vi "PositionCtrl_TurnToAngle_Example.vi"() -> ()   [LabVIEW 2019]
uses:
  <vilib>/Rock Robotics/WPI/ThirdParty/JAS_Junk/TrajLib/SlewRateLimiter_New.vi
  <vilib>/Rock Robotics/WPI/ThirdParty/JAS_Junk/TrajLib/SlewRateLimiter_Reset.vi
  <vilib>/Rock Robotics/WPI/ThirdParty/JAS_Junk/TrajLib/SlewRateLimiter_Calculate.vi
  <vilib>/Rock Robotics/WPI/ThirdParty/JAS_Junk/TrajLib/SlewRateLimiter_SetRate.vi
  <vilib>/Rock Robotics/WPI/ThirdParty/JAS_Junk/TrajLib/Util_GetTime.vi
  <vilib>/Rock Robotics/WPI/ThirdParty/JAS_Junk/TrajLib/VI/Util_GetTime_U32.vi
  <vilib>/Rock Robotics/WPI/ThirdParty/JAS_Junk/TrajLib/VI/Util_GetTime_U64.vi
  <vilib>/Rock Robotics/WPI/ThirdParty/JAS_Junk/TrajLib/Trajectory_Library.lvlib
panel:
  in  "Tab Control":enum32{"Operation", "Tuning"}(tab)
  out "Targets along the way":cluster{dbl, "PositionError":dbl, "modulus":dbl}(graph)
  in  "SP - Desired Angle\n (Deg)":dbl(slide) scale=-10.0..350.0
  out "PV - Current Angle\n (Deg)":dbl(slide) scale=-10.0..350.0
  out "Goal Chart":T1(graph)
  out "Motor Output":dbl format="%13.3f"
  out "Within Deadband":bool
  out "PositionError  (Deg)":dbl format="%13.2f"
  out "Velocity  (Deg/Sec)":dbl format="%13.2f"
  in  "Output Threshold":dbl=1.0 format="%#_13g"
  in  "Output Deadband":dbl=0.08 format="%#_13g"
  in  "Max Motor Output (+/-1)":dbl=1.0 format="%#_13g"
  in  "Error Tolerance\n(Deg)":dbl=0.5 format="%#_13g"
  in  "Error Threshold\n(Deg)":dbl=25.0 format="%#_13g"
  in  "At Reference Count":i32=13
  # "PID Tuning Parameters"
  # "Desired Profile Performance"
  # "Desired On Target Tolerance"
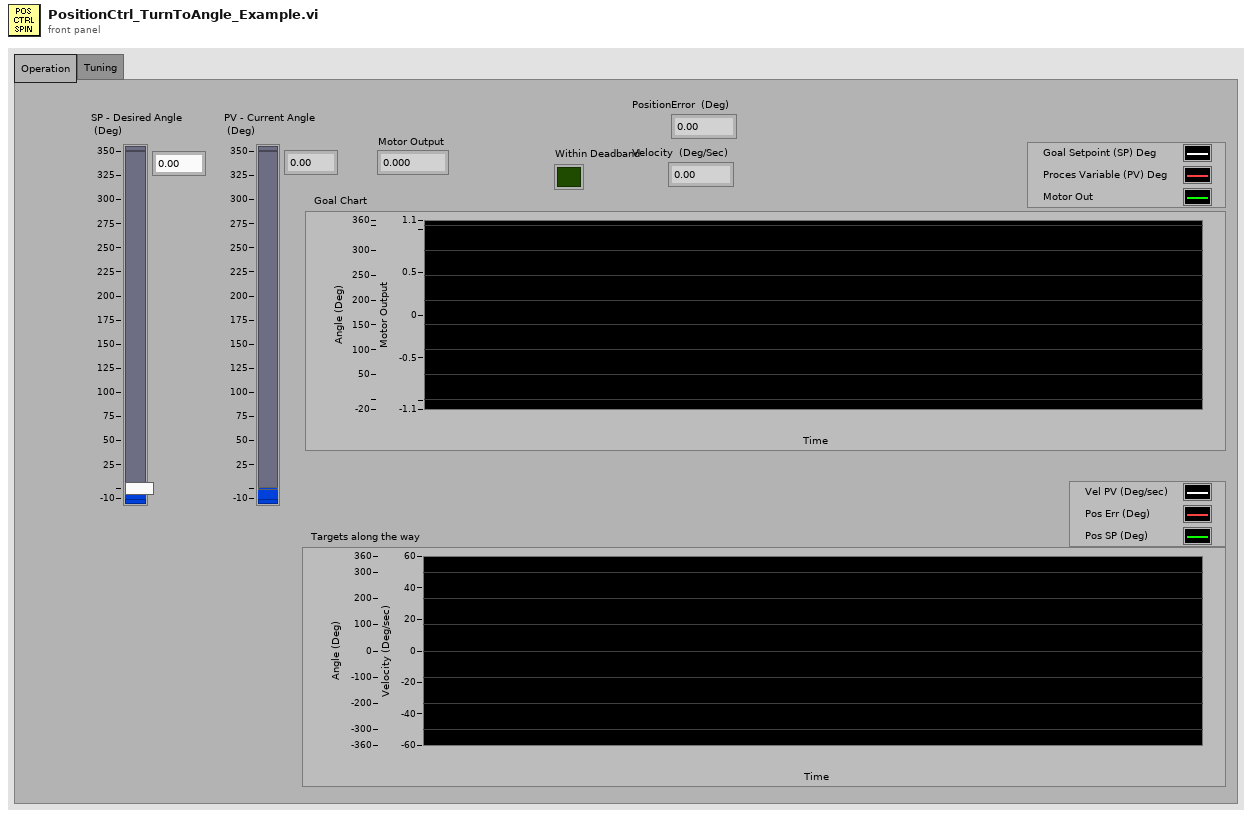
[diagram p1: front panel]
types:
  T1 = cluster{"SP - Desired Position\n (Inch)":dbl, "upper limit":dbl, "upper limit":dbl}
  T2 = typedef "Trajectory_Library.lvlib/PosCtrl_Tuning_Type.ctl" = cluster{"Slope":dbl, "Offset":dbl, "Error Deadband":dbl, "At Reference Count":i32, "Negate Output":bool, "Max Allowd Position":dbl, "Min Allowd Position":dbl}
  T3 = cluster{"SP - Desired Angle\n (Deg)":dbl, "modulus":dbl, "Result":dbl}
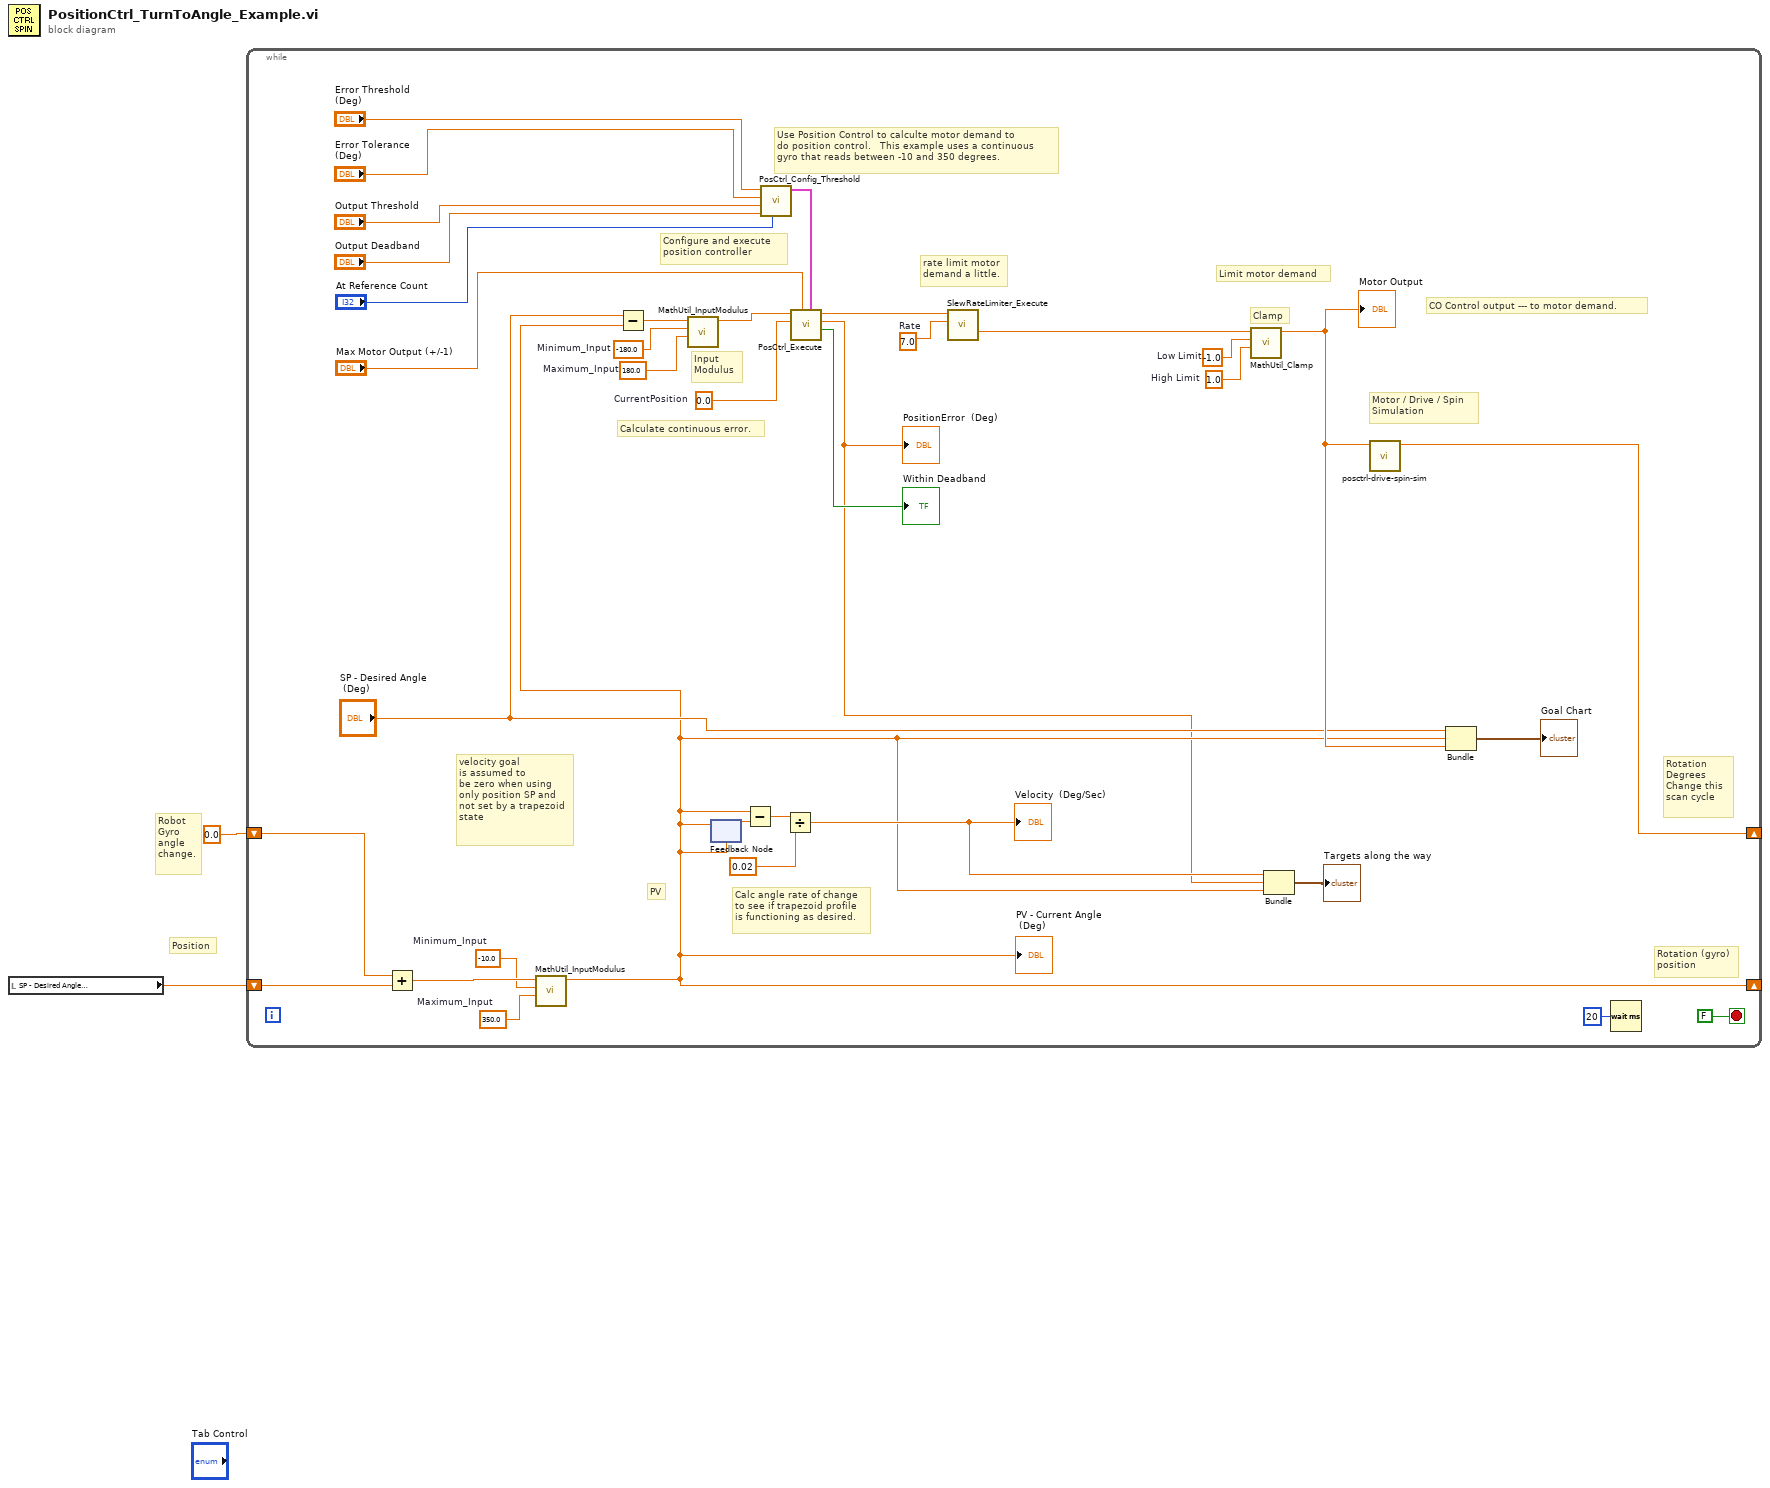
[diagram p0: block diagram]
diagram:
  # "Position"
  # "Robot\nGyro\nangle\nchange."
  n1 = local read "SP - Desired Angle\n (Deg)"() -> (w1:dbl)
  n2 = while {
    shift-right: [w12] -> _
    shift-left: w1 -> [w32]
    shift-right: [w26] -> _
    shift-left: 0.0 ("upper limit") -> [w27]
    stop <- FALSE stop-if-true
    w15 = -180.0  # Minimum_Input
    w17 = 180.0  # Maximum_Input
    w25 = 0.0  # CurrentPosition
    w21 = 1.0  # High Limit
    w20 = -1.0  # Low Limit
    w23 = 7.0  # Rate
    w28 = -10.0  # Minimum_Input
    w29 = 350.0  # Maximum_Input
    # "Calculate continuous error."
    # "rate limit motor\ndemand a little."
    # "Input\nModulus"
    # "Clamp"
    # "Configure and execute \nposition controller"
    # "Use Position Control to calculte motor demand to\ndo position control.   This example uses a continuous\ngyro that reads between -10 and 350 degrees."
    # "Rotation (gyro)\nposition"
    # "Rotation\nDegrees \nChange this \nscan cycle"
    # "CO Control output --- to motor demand."
    # "Motor / Drive / Spin\nSimulation"
    # "Limit motor demand"
    # "PV"
    # "Calc angle rate of change\nto see if trapezoid profile\nis functioning as desired."
    # "velocity goal\nis assumed to \nbe zero when using\nonly position SP and\nnot set by a trapezoid\nstate"
    n3 = Add(x=w27, y=w32) -> (x+y=w30:dbl)
    n4 = call <vilib>:"MathUtil_InputModulus.vi"("Maximum_Input"=w29, "Minimum_Input"=w28, "Input"=w30) -> ("modulus"=w12:dbl)  [unwired: 8 in]
    "PV - Current Angle\n (Deg)" <- w12
    n5 = Subtract(x="SP - Desired Angle\n (Deg)", y=w12) -> (x-y=w14:dbl)
    n6 = call <vilib>:"MathUtil_InputModulus.vi"("Maximum_Input"=w17, "Minimum_Input"=w15, "Input"=w14) -> ("modulus"=w16:dbl)  [unwired: 8 in]
    n7 = feedback-in #1(w12) -> ()
    n8 = feedback #1(w12) -> (w36:dbl)
    n9 = Subtract(x=w12, y=w36) -> (x-y=w35:dbl)
    n10 = call <vilib>:"PosCtrl_Config_Threshold.vi"("At Reference Count"="At Reference Count", "Output Deadband"="Output Deadband", "Output Threshold"="Output Threshold", "ErrorDeadband"="Error Tolerance\n(Deg)", "ErrorThreshold"="Error Threshold\n(Deg)") -> ("PosCtrl_Config_Params"=w24:T2)  [unwired: 6 in]
    n11 = Divide(x=w35, y=0.02) -> (x/y=w31:dbl)
    "Velocity  (Deg/Sec)" <- w31
    n12 = call <vilib>:"PosCtrl_Execute.vi"("PosCtrl_Config_Params"=w24, "MaxOutput"="Max Motor Output (+/-1)", "CurrentPosition"=w25, "TargetPosition"=w16) -> ("OnTarget"=→"Within Deadband":bool, "PositionError"=w4:dbl, "Output"=w22:dbl)  [unwired: 5 in]
    "PositionError  (Deg)" <- w4
    n13 = call <vilib>:"SlewRateLimiter_Execute.vi"("PositiveRate"=w23, "Input"=w22) -> ("Output"=w19:dbl)  [unwired: 8 in, 1 out]
    n14 = call <vilib>:"MathUtil_Clamp.vi"("High Limit"=w21, "Low Limit"=w20, "Value"=w19) -> ("Result"=w18:dbl)  [unwired: 8 in]
    "Motor Output" <- w18
    n15 = Bundle(w31, "PositionError"=w4, "modulus"=w12) -> (→"Targets along the way":cluster{dbl, "PositionError":dbl, "modulus":dbl})  [unwired: 1 in]
    n16 = call "posctrl-drive-spin-sim.vi"("Motor Demand"=w18) -> ("Rotation Change Deg"=w26:dbl)  [unwired: 10 in]
    n17 = Bundle("SP - Desired Angle\n (Deg)"="SP - Desired Angle\n (Deg)", "modulus"=w12, "Result"=w18) -> (→"Goal Chart":T3)  [unwired: 1 in]
    n18 = Wait (ms)(milliseconds to wait=u32 20) -> ()  [unwired: 1 out]
  }
